vi "Data Log Overwrite Warning.vi"(8 "error in (no error)":errorcluster, 11 "Settings in":T1) -> (0 "error out":errorcluster, 2 "Overwrite Warning?":bool, 3 "Settings out":T1)   [LabVIEW 2021, in "Settings.lvlib"]
doc: "If the Log.Path from 'Settings in' exists and Log.Append? is FALSE, then indicate that the data log file will be overwritten in 'Overwrite Warning?'"
uses:
  Settings.lvlib
  Acquisition/IO Device.ctl
  Acquisition/Acquisition.lvlib
  Acquisition/Channel Settings.ctl
  Interval Timer/Interval Length.ctl
  Interval Timer/Interval Timer.lvlib
  Interval Timer/Repeat Interval.ctl
  Interval Timer/Interval Token.ctl
  Acquisition/Hardware Configuration.ctl
  Logging/Logging Configuration.ctl
  Logging/Logging.lvlib
  Diagnostics/Diagnostics Configuration.ctl
  Diagnostics/Diagnostics.lvlib
  Settings.ctl
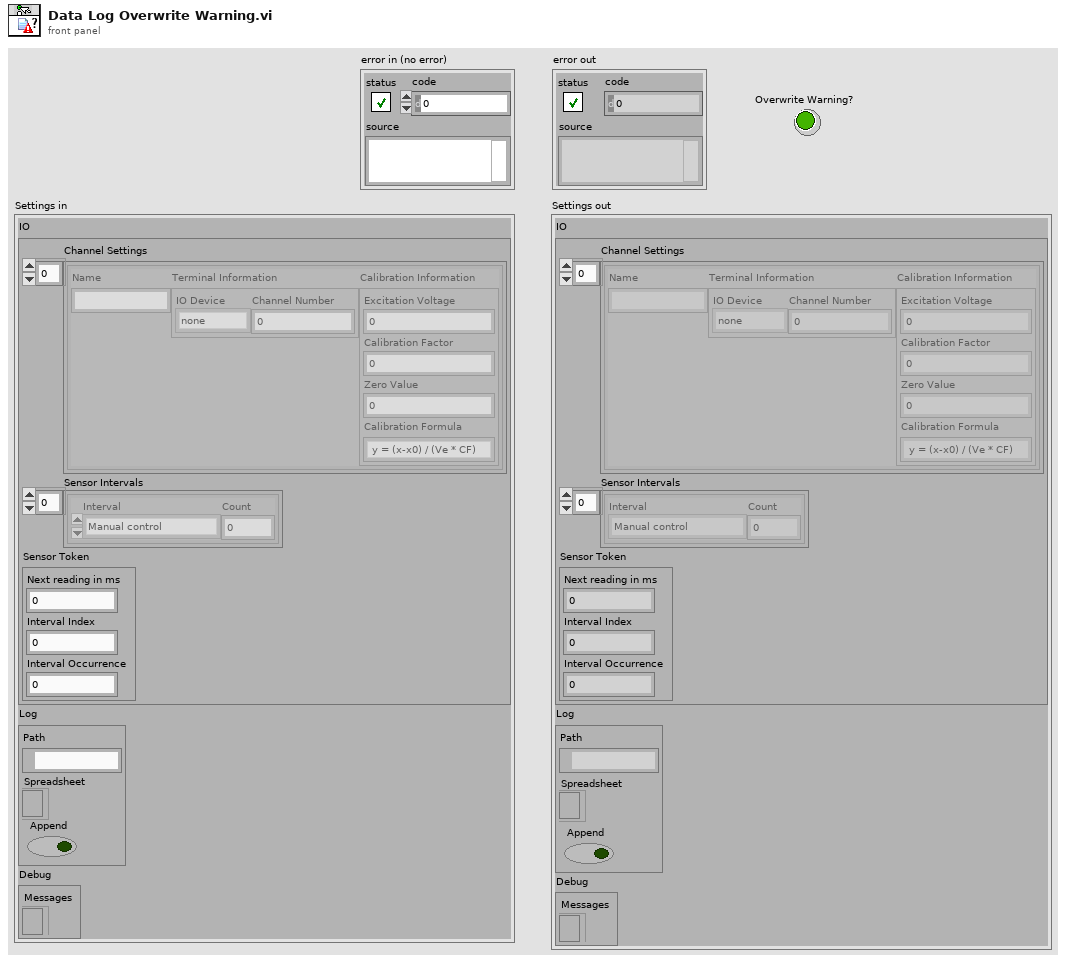
[diagram p1: front panel]
types:
  T1 = typedef "Settings.lvlib/Settings.ctl" = cluster{"IO":T2, "Log":T8, "Debug":T9}
  T2 = typedef "Acquisition.lvlib/Hardware Configuration.ctl" = cluster{"Channel Settings":T3[], "Sensor Intervals":T5[], "Sensor Token":T7}
  T3 = typedef "Acquisition.lvlib/Channel Settings.ctl" = cluster{"Name":string, "Terminal Information":cluster{"IO Device":T4, "Channel Number":i32}, "Calibration Information":cluster{"Excitation Voltage":dbl, "Calibration Factor":dbl, "Zero Value":dbl, "Calibration Formula":string}}
  T4 = typedef "Acquisition.lvlib/IO Device.ctl" = enum16{"none", "9219", "9401"}
  T5 = typedef "Interval Timer.lvlib/Repeat Interval.ctl" = cluster{"Interval":T6, "Count":i32}
  T6 = typedef "Interval Timer.lvlib/Interval Length.ctl" = enum16{"Manual control", "1 second", "10 seconds", "30 seconds", "60 seconds", "600 seconds", "1200 seconds", "3600 seconds"}
  T7 = typedef "Interval Timer.lvlib/Interval Token.ctl" = cluster{"Next reading in ms":u32, "Interval Index":i32, "Interval Occurrence":i32}
  T8 = typedef "Logging.lvlib/Logging Configuration.ctl" = cluster{"Path":path, "Spreadsheet":refnum<file>, "Append":bool}
  T9 = typedef "Diagnostics.lvlib/Diagnostics Configuration.ctl" = cluster{"Messages":refnum<file>}
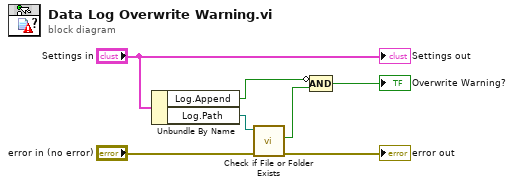
[diagram p0: block diagram]
diagram:
  n1 = Unbundle By Name("Settings in") -> ("Log.Append"=w5:bool, "Log.Path"=w7:path)
  n2 = call <vilib>:"Check if File or Folder Exists.vi"("error in (no error)"="error in (no error)", "path"=w7) -> ("error out"=→"error out":errorcluster, "file or folder exists?"=w6:bool)  [unwired: 7 in, 1 out]
  n3 = Compound Arithmetic op=AND(invert w5, w6) -> (→"Overwrite Warning?":bool)
  "Settings out" <- "Settings in"
